vi "Read Dual Fan Actor.vi"(11 "Evaporative Cooler":refnum<class "Evaporative Cooler.lvclass">) -> (2 "Dual Fan":refnum<class "Dual Fan.lvclass">)   [LabVIEW 2025, in "Evaporative Cooler.lvlib" / "Evaporative Cooler.lvclass"]
doc: "Read the Dual Fan actor that should be launched by this Evaporative Cooler. Child classes should override this method to return the Dual Fan that best meets their needs. For example, a simulated evaporative cooler would return a simulated dual fan."
uses:
  Evaporative Cooler.lvclass
  Dual Fan/Dual Fan/Dual Fan.lvclass
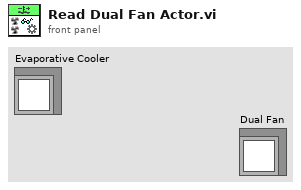
[diagram p1: front panel]
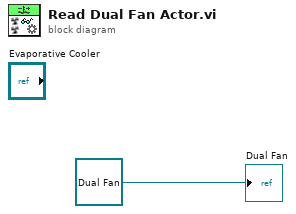
[diagram p0: block diagram]
diagram:
  "Dual Fan" <- refnum<class "Dual Fan.lvclass"> refnum ("Dual Fan.lvclass")
